vi "Read Next Empty Row.vi"(8 "error in (no error)":errorcluster, 11 "Excel Sheet in":refnum<class "Excel Sheet.lvclass">) -> (0 "error out":errorcluster, 2 "Next Empty Row":i32, 3 "Excel Sheet out":refnum<class "Excel Sheet.lvclass">)   [LabVIEW 2013, in "Excel Sheet.lvclass"]
uses:
  Excel Sheet.lvclass
  Excel Sheet.lvclass/Excel Sheet.ctl
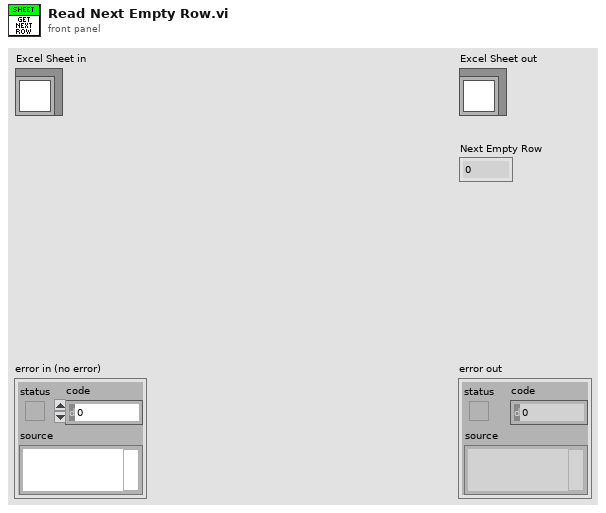
[diagram p1: front panel]
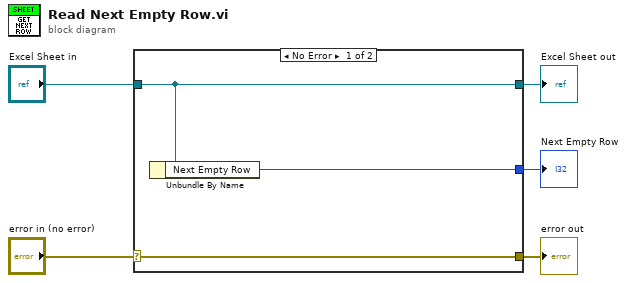
[diagram p0: block diagram]
diagram:
  n1 = case shown="No Error" "error in (no error)" {
    selector: "error in (no error)" -> [w8 w9]
    tunnel: [w8 w9] -> w4
    tunnel: [w7 w10] -> w2
    tunnel: "Excel Sheet in" -> [w7 w10]
    tunnel: [w6 _] -> w1
    frame No Error {
      n2 = Unbundle By Name(w7) -> ("Next Empty Row"=w6:i32)
    }
    frame Error {
    }
  }
  "error out" <- w4
  "Excel Sheet out" <- w2
  "Next Empty Row" <- w1
